vi "nosync1.vi"(5 "h 2":waveform(i16)[](array[waveform])) -> (1 "h 3":waveform(i16)[](array[waveform]))   [LabVIEW 2010]
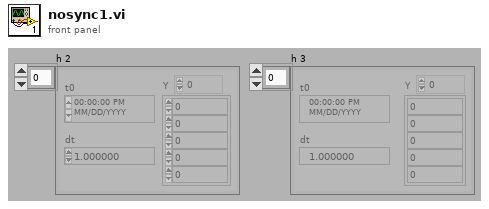
[diagram p1: front panel]
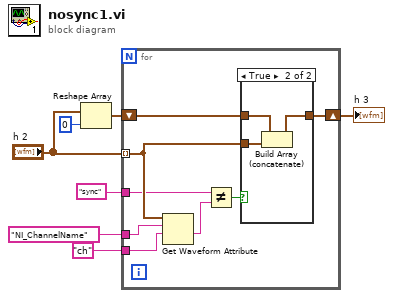
[diagram p0: block diagram]
diagram:
  n1 = Reshape Array("h 2", 0 ("dimension size")) -> (w6:waveform(i16)[])
  n2 = for {
    tunnel: "h 2" -> [w11] mode=indexing
    shift-right: [w12] -> w4
    shift-left: w6 -> [w13]
    tunnel: "NI_ChannelName" ("name") -> [w10]
    tunnel: "ch" ("name") -> [w9]
    tunnel: "sync" ("x") -> [w8]
    n3 = Get Waveform Attribute(5:w9, 6:w10, 7:w11) -> (1:w15:string)  [unwired: 1 in, 3 out]
    n4 = Not Equal?(x=w8, y=w15) -> (x != y?=w14:bool)
    n5 = case shown="True" w14 {
      tunnel: w13 -> [w16 w19]
      tunnel: [w16 w18] -> w12
      tunnel: w11 -> [_ w17]
      frame False {
      }
      frame True {
        n6 = Build Array (concatenate)(w19, w17) -> (w18:waveform(i16)[])
      }
    }
  }
  "h 3" <- w4
